vi "Connect.vi"(8 "error in (no error)":errorcluster, 9 "Custom Connection Data":variant, 10 "Connection Name":string, 11 "RTFIFODouble in":refnum<class "CIFTag.lvclass">) -> (0 "error out":errorcluster, 3 "RTFIFODouble out":refnum<class "CIFTag.lvclass">)   [LabVIEW 2021, in "CIFTag.lvclass"]
uses:
  CIFTag.lvclass
  D:/dev/CIF-LVCore/src/CIFUtilities/CIFChannels/CIFChannels.lvclass
  CIFUtilities/CIFChannels/Typedef/Channel State.ctl
  CIFUtilities/CIFChannels/CIFChannels.lvclass/CIFChannels.ctl
  CIFTag.lvclass/CIFTag.ctl
  CIFUtilities/CIFChannels/Accessors/Write Channel State.vi
  CIFUtilities/CIFChannels/CIFChannels.lvclass
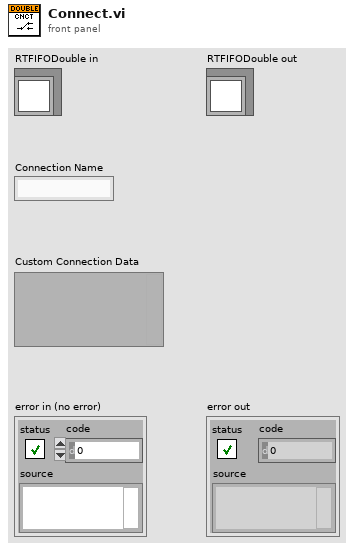
[diagram p1: front panel]
types:
  T1 = typedef "CIFChannels.lvclass/Channel State.ctl" = enum16{"Creating", "Disconnected", "Connecting", "Connected", "Destroying"}
  T2 = cluster{"read mode":enum16{"polling", "blocking"}, "write mode":enum16{"polling", "blocking"}}
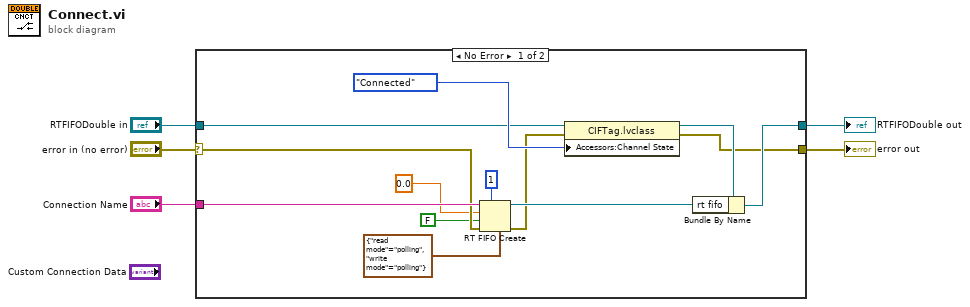
[diagram p0: block diagram]
diagram:
  n1 = case shown="No Error" "error in (no error)" {
    selector: "error in (no error)" -> [w9 w20]
    tunnel: [w10 w20] -> w4
    tunnel: [w14 w19] -> w2
    tunnel: "RTFIFODouble in" -> [w8 w19]
    tunnel: "Connection Name" -> [w18 _]
    frame No Error {
      n2 = RT FIFO Create(0:w18, 1:0.0, 2:FALSE ("create if not found? (T)"), 3:w9, 4:u32 1 ("size (10)"), 7:T2 {"read mode"=enum."polling", "write mode"=enum."polling"} ("r/w modes (polling,polling)")) -> (8:w15:refnum<k33>, 11:w11:errorcluster)  [unwired: 2 in, 1 out]
      n3 = property class="CIFTag.lvclass"(reference=w8, error in=w11, "Accessors:Channel State"=Channel_State."Connected" ("Channel State")) -> (reference out=w13:refnum<class "CIFTag.lvclass">, error out=w10:errorcluster)
      n4 = Bundle By Name(cluster=w13, "rt fifo"=w15) -> (w14:refnum<class "CIFTag.lvclass">)
    }
    frame Error {
    }
  }
  "error out" <- w4
  "RTFIFODouble out" <- w2
